vi "FieldSweepScans.vi"() -> ()   [LabVIEW 2021]
uses:
  <instrlib>/Zurich Instruments LabOne/Public/Configure/ziSetValueDoubleArray.vi
  <instrlib>/Zurich Instruments LabOne/Public/Configure/ziSetValueDouble.vi
  <instrlib>/Zurich Instruments LabOne/Public/Configure/ziGetValueDemodSampleEx.vi
  <instrlib>/Zurich Instruments LabOne/Zurich Instruments LabOne.lvlib
panel:
  in  "Tab Control 2":enum32{"Measurement OP"}(tab)
  in  "ms time per field OP":dbl=500.0
  in  "Max OP voltage":dbl
  in  "Min OP voltage":dbl
  in  "Delta OP voltage":dbl=0.25
  in  "N.Loops OOP":i32
  in  "N. measures OP":dbl=1.0
  in  "ms time mes. OP":dbl=500.0
  out "Current OOP":cluster{dbl[], dbl[]}(graph)
  in  "Measure OP":bool
  out "Average OOP":cluster{dbl[], dbl[]}(graph)
  out "OP loop":i32
  in  "stop":bool
  in  "Try IP voltage":enum32{"Single Voltage Output"}(tab)
  in  "OP voltage":dbl
  in  "IP voltage":dbl
  in  "In Plane":bool
  in  "Out Plane":bool
  in  "Tab Control":enum32{"Measurement IP"}(tab)
  in  "Measure IP":bool
  in  "ms time mes. IP":dbl=500.0
  in  "Min IP voltage":dbl
  in  "Delta IP voltage":dbl=0.25
  in  "Max IP voltage":dbl
  in  "N. measures IP":dbl=1.0
  in  "ms time per delta":dbl=500.0
  in  "Loops IP":i32
  out "Current IP":cluster{dbl[], dbl[]}(graph)
  out "Updated IP":cluster{dbl[], dbl[]}(graph)
  out "IP loop":i32
  in  "Lock-In Parameters Tab":enum32{"Lock-In Parameters IP"}(tab)
  in  "Frequency (Hz)":dbl=1092.0
  in  "Harm.":u32=1
  in  "Order 1":enum16{"1", "2", "3", "4", "5", "6", "7", "8"}(ring)=enum."6" caption="Order"
  in  "TC Value 1":dbl=68.99 caption="Value (s/Hz)" format="%#_8g"
  in  "TC/BW 1":enum16{"TC", "BW 3dB"}(ring)=enum."BW 3dB" caption="TC/BW"
  in  "Vpeak (V)":dbl
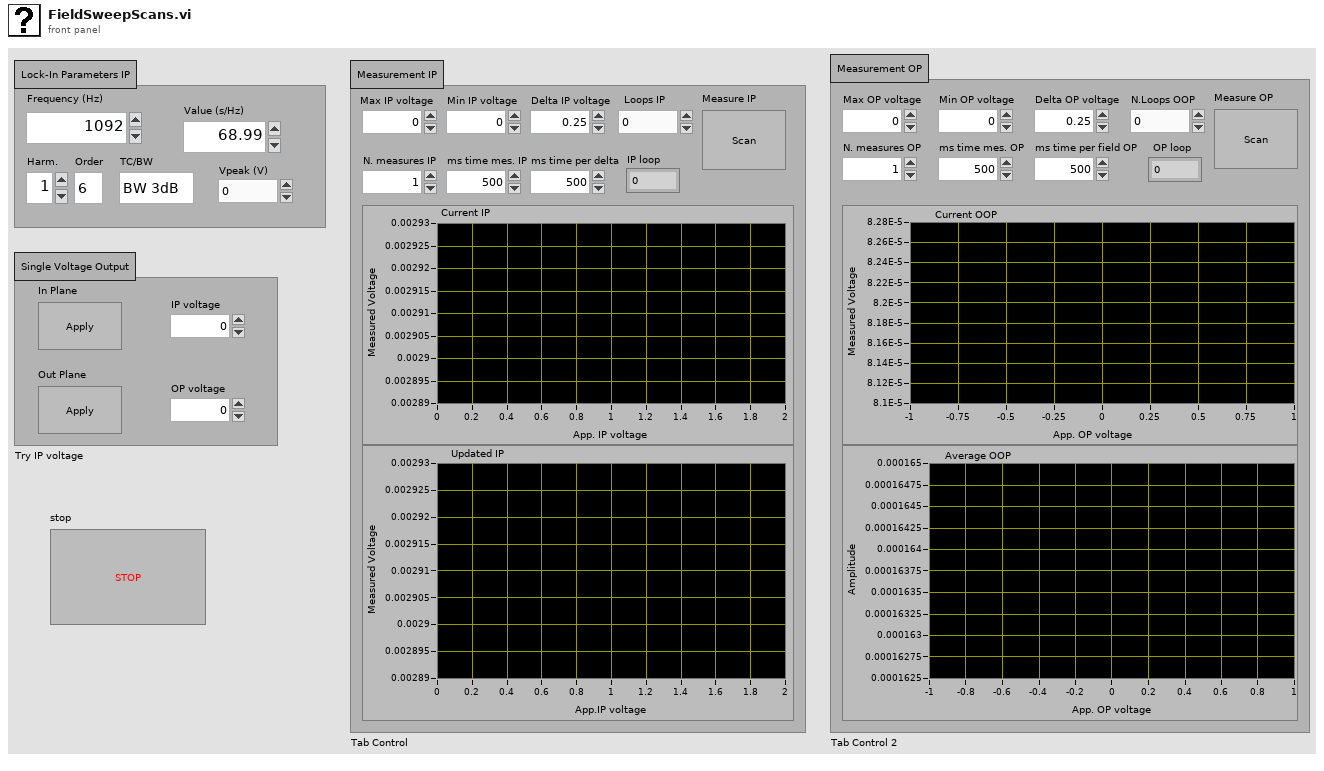
[diagram p1: front panel]
types:
  T1 = typedef "Zurich Instruments LabOne.lvlib/ziTypeHandle.ctl" = cluster{"handleValid":bool, "Conn":u64, "Path Prefix":string, "Handle":u64, "Connected":bool, "Clockbase(s)":dbl}
  T2 = typedef "Zurich Instruments LabOne.lvlib/ziTypeDemodSampleSingle.ctl" = cluster{"Timestamps (ticks)":u64, "X (Vrms)":dbl, "Y (Vrms)":dbl, "Osc Phase (deg)":dbl, "Freq (Hz)":dbl, "DIO":u32, "AuxIn0 (V)":dbl, "AuxIn1 (V)":dbl, "Trigger":u32}
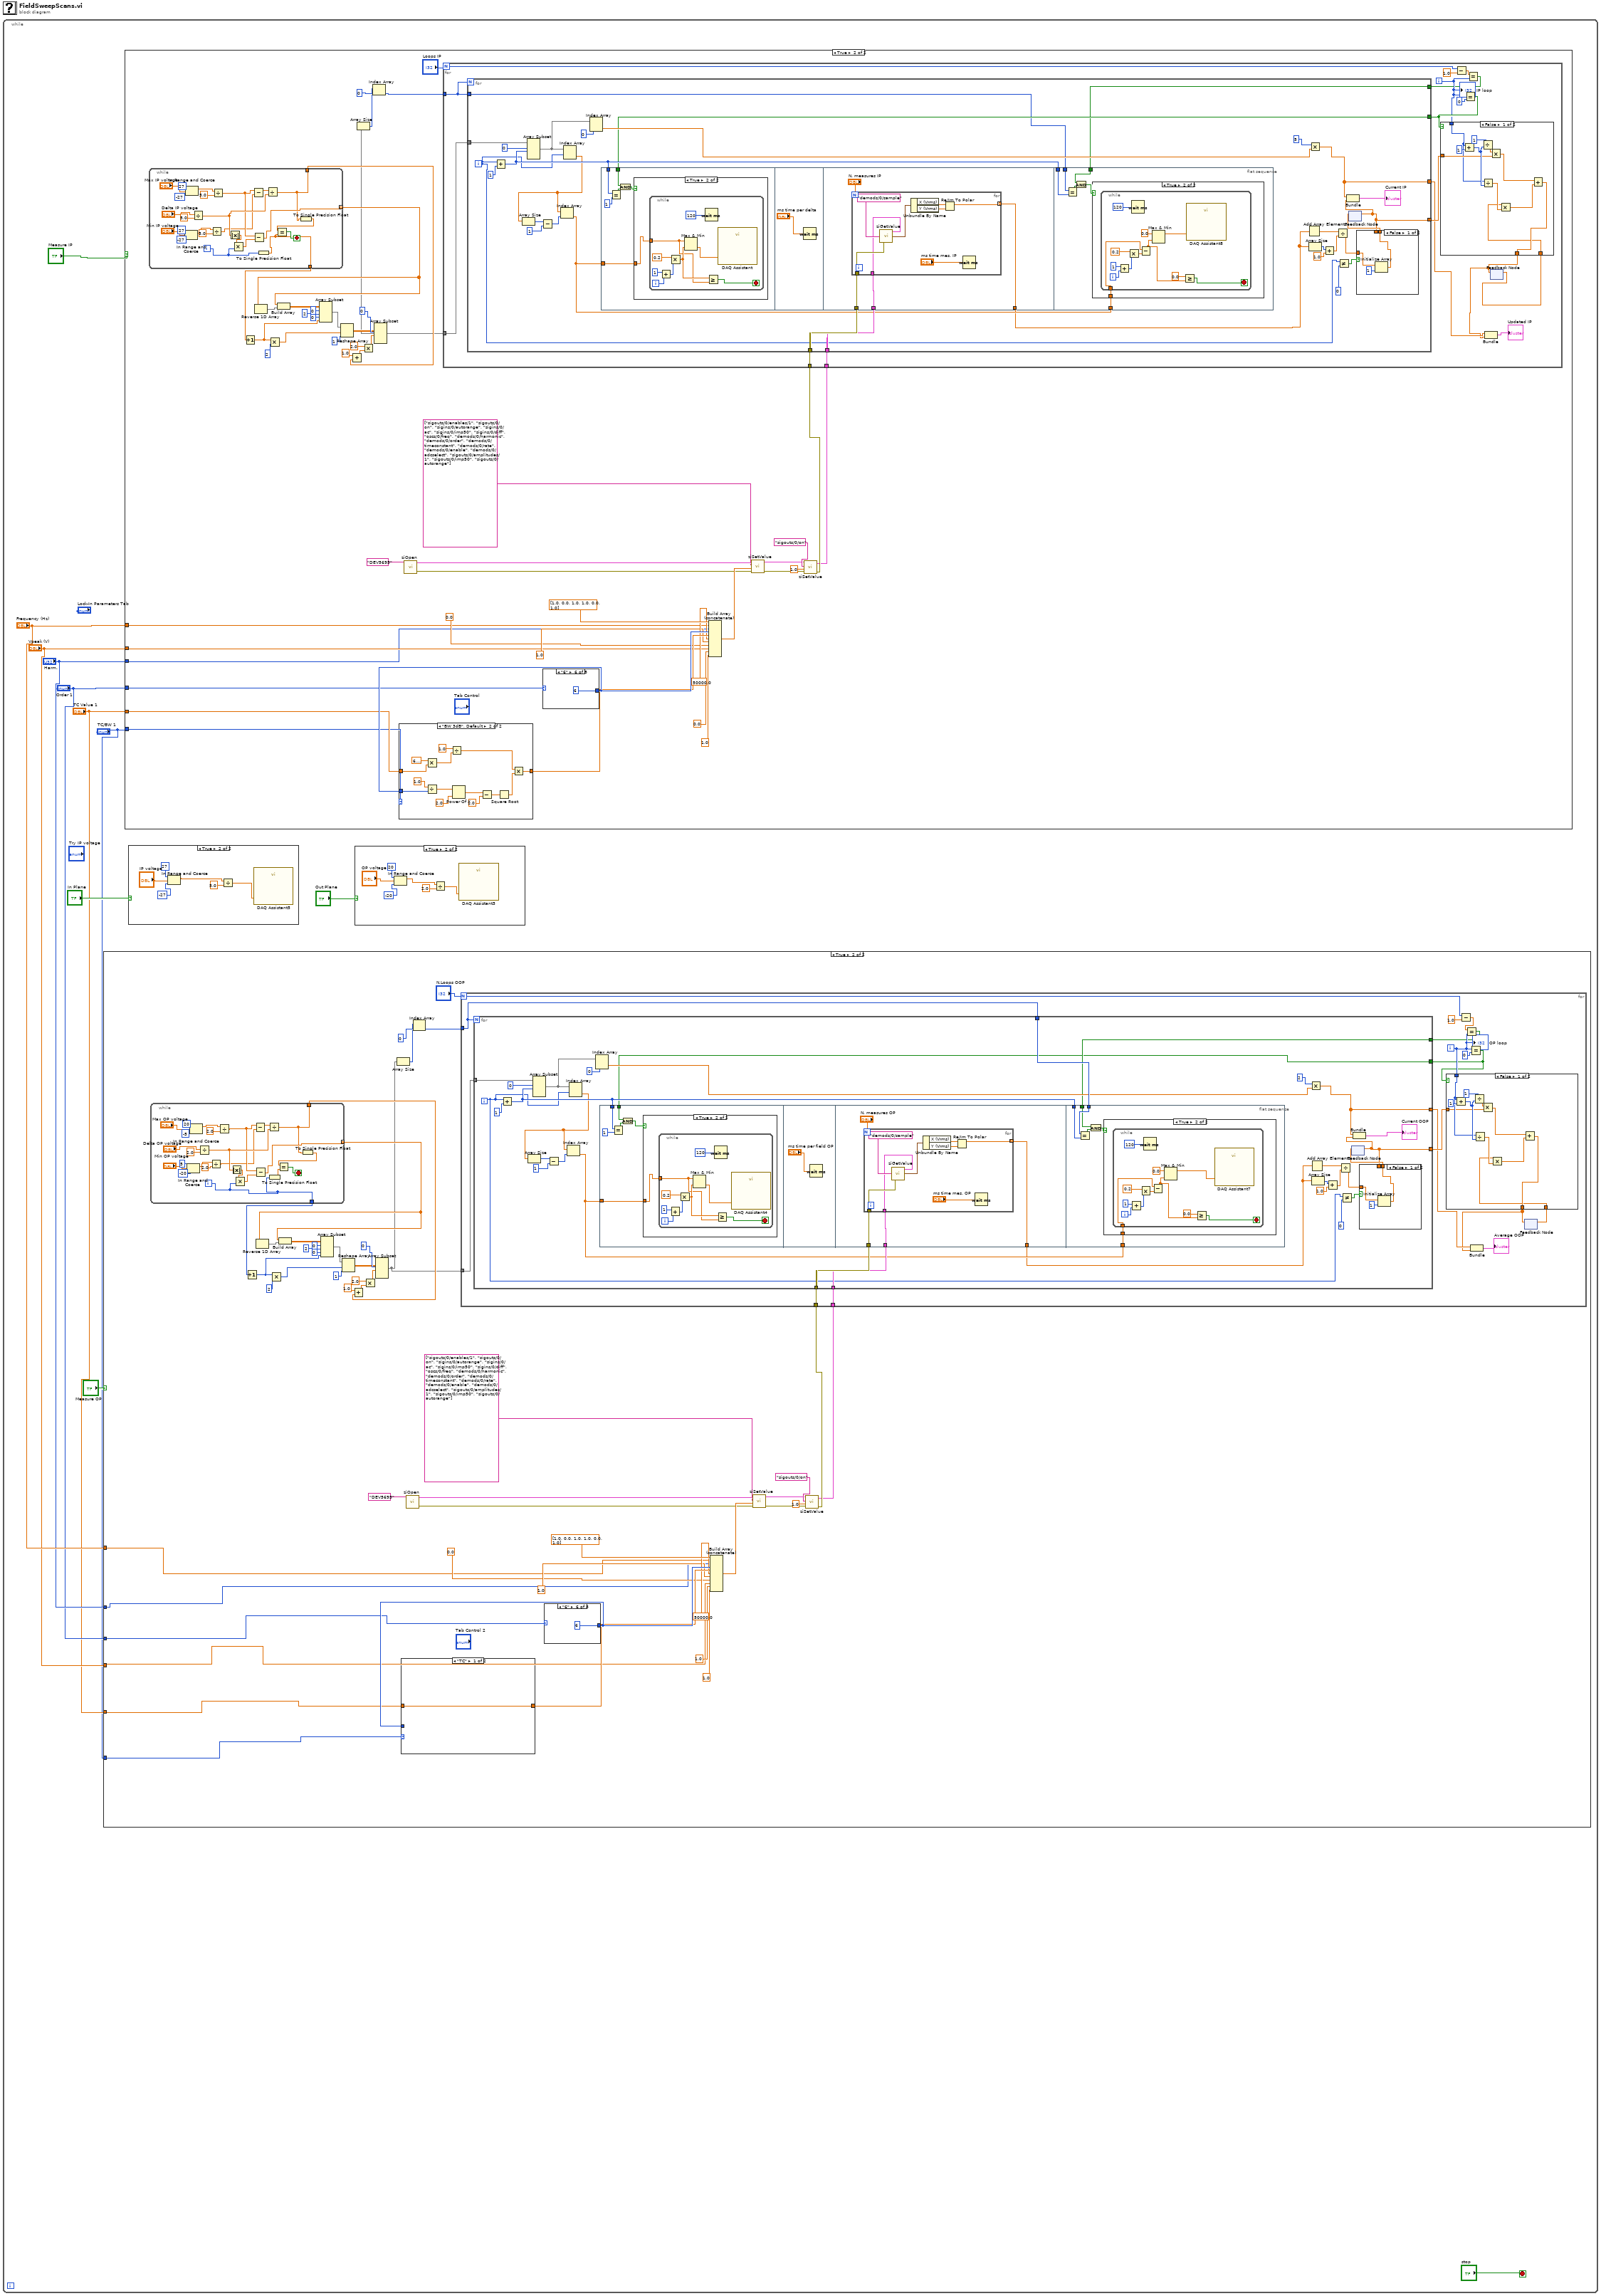
[diagram p0: block diagram]
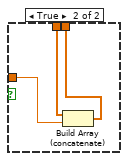
[diagram p4: hidden frame]
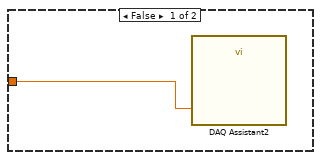
[diagram p5: hidden frame]
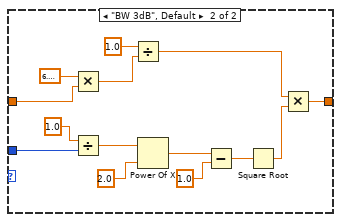
[diagram p7: hidden frame]
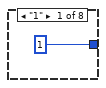
[diagram p8: hidden frame]
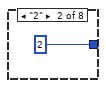
[diagram p9: hidden frame]
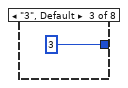
[diagram p10: hidden frame]
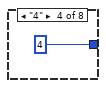
[diagram p11: hidden frame]
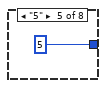
[diagram p12: hidden frame]
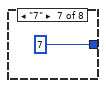
[diagram p13: hidden frame]
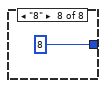
[diagram p14: hidden frame]
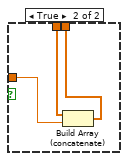
[diagram p19: hidden frame]
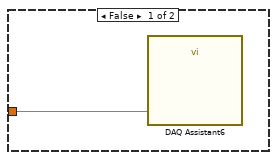
[diagram p20: hidden frame]
diagram:
  n1 = while {
    stop <- "stop" stop-if-true
    n2 = case shown="True" "Measure OP" {
      tunnel: "Frequency (Hz)" -> [_ w18]
      tunnel: "Vpeak (V)" -> [_ w17]
      tunnel: "Harm." -> [_ w16]
      tunnel: "Order 1" -> [_ w15]
      tunnel: "TC Value 1" -> [_ w14]
      tunnel: "TC/BW 1" -> [_ w13]
      frame False {
      }
      frame True {
        n3 = while {
          tunnel: [w194] -> w41 mode=indexing
          tunnel: [w178] -> w38
          tunnel: [w177] -> w33
          i -> [w178]
          stop <- w197 stop-if-true
          n4 = In Range and Coerce(upper limit=5, x="Min OP voltage", lower limit=-20) -> (coerced(x)=w181:dbl)  [unwired: 1 out]
          n5 = In Range and Coerce(upper limit=20, x="Max OP voltage", lower limit=-5) -> (coerced(x)=w183:dbl)  [unwired: 1 out]
          n6 = Divide(x="Delta OP voltage", y=2.0) -> (x/y=w189:dbl)
          n7 = Divide(x=w181, y=2.0) -> (x/y=w179:dbl)
          n8 = Divide(x=w183, y=2.0) -> (x/y=w180:dbl)
          n9 = Absolute Value(x=w189) -> (abs(x)=w196:dbl)
          n10 = Multiply(x=w196, y=w178) -> (x*y=w195:dbl)
          n11 = Subtract(x=w180, y=w179) -> (x-y=w198:dbl)
          n12 = Subtract(x=w180, y=w195) -> (x-y=w194:dbl)
          n13 = Divide(x=w198, y=w189) -> (x/y=w177:dbl)
          n14 = To Single Precision Float(number=w178) -> (single precision float=w176:sgl)
          n15 = To Single Precision Float(number=w177) -> (single precision float=w175:sgl)
          n16 = Equal?(x=w175, y=w176) -> (x = y?=w197:bool)
        }
        n17 = Increment(x=w38) -> (x+1=w22:i32)
        n18 = Reverse 1D Array(array=w41) -> (reversed array=w40:dbl[])
        n19 = Multiply(x=w22, y=2) -> (x*y=w24:i32)
        n20 = Build Array "Build Array"(w41, w40) -> (w21:dbl[][])
        n21 = Array Subset(array=w21, index (row)=0 ("index"), length (row)=2 ("length"), index (col)=0 ("index"), length (col)=w22) -> (w20:dbl[][])
        n22 = Reshape Array(w20, w24, 1 ("dimension size")) -> (w27:dbl[][])
        n23 = Add(x=1.0, y=w33) -> (x+y=w31:dbl)
        n24 = Multiply(x=2.0, y=w31) -> (x*y=w30:dbl)
        n25 = Array Subset(array=w27, index (row)=0 ("index"), length (row)=w30) -> (w28:dbl[][])  [unwired: 2 in]
        n26 = Array Size(array=w28) -> (size(s)=w35:i32[])
        n27 = call <instrlib>:"ziOpen.vi"("Address"="DEV5695") -> ("Error Out"=w57:errorcluster, "HandleOut"=w56:T1)  [unwired: 3 in, 1 out]
        n28 = Index Array(array=w35, index=0) -> (element=w12:i32)
        n29 = case shown="\"6\"" w15 {
          tunnel: [1 2 3 4 5 6 7 8] -> w59
          frame "1" {
          }
          frame "2" {
          }
          frame "3", Default {
          }
          frame "4" {
          }
          frame "5" {
          }
          frame "6" {
          }
          frame "7" {
          }
          frame "8" {
          }
        }
        n30 = case shown="\"TC\"" w13 {
          tunnel: w14 -> [w199 w202]
          tunnel: [w199 w201] -> w58
          tunnel: w59 -> [_ w200]
          frame "TC" {
          }
          frame "BW 3dB", Default {
            n31 = Multiply(x=6.283185307179586, y=w202) -> (x*y=w211:dbl)
            n32 = Divide(x=1.0, y=w200) -> (x/y=w204:dbl)
            n33 = Divide(x=1.0, y=w211) -> (x/y=w208:dbl)
            n34 = Power Of X(1:2.0 ("x"), 2:w204) -> (0:w205:dbl)
            n35 = Subtract(x=w205, y=1.0) -> (x-y=w209:dbl)
            n36 = Square Root(x=w209) -> (sqrt(x)=w207:dbl)
            n37 = Multiply(x=w208, y=w207) -> (x*y=w201:dbl)
          }
        }
        n38 = Build Array (concatenate) "Build Array"(dbl[] [1.0, 0.0, 1.0, 1.0, 0.0, 1.0], w18, w16, w59, w58, 50000.0 ("t"), 1.0 ("t"), 0.0 ("element"), w17, 1.0 ("element"), 1.0 ("element")) -> (w60:dbl[])
        n39 = call-poly <instrlib>:"ziSetValue.vi"("Error In"=w57, "Values"=w60, "Paths"=string[] ["sigouts/0/enables/1", "sigouts/0/on", "sigins/0/autorange", "sigins/0/ac", "sigins/0/imp50", "sigins/0/diff", "oscs/0/freq", "demods/0/harmonic", "demods/0/order", "demods/0/timeconstant", "demods/0/rate", "demods/0/enable", "demods/0/adcselect", "sigouts/0/amplitudes/1", "sigouts/0/imp50", "sigouts/0/autorange"], "Handle In"=w56) -> ("Error Out"=w44:errorcluster, "Handle Out"=w45:T1)  [unwired: 1 in]
        n40 = call-poly <instrlib>:"ziSetValue.vi"("Error In"=w44, "Value"=1.0, "Path"="sigouts/0/on", "Handle In"=w45) -> ("Error Out"=w43:errorcluster, "Handle Out"=w42:T1)  [unwired: 1 in]
        n41 = for {
          N: "N.Loops OOP" -> [w69]
          tunnel: w43 -> [w76]
          tunnel: w42 -> [w75]
          tunnel: w12 -> [w73]
          tunnel: w28 -> [w74]
          i -> [w68]
          n42 = Subtract(x=w69, y=1.0) -> (x-y=w67:dbl)
          n43 = Equal?(x=w67, y=w68) -> (x = y?=w66:bool)
          n44 = Equal?(x=w68, y=0) -> (x = y?=w61:bool)
          n45 = for {
            N: w73 -> [_]
            tunnel: w76 -> [w119]
            tunnel: w75 -> [w118]
            tunnel: w74 -> [w115]
            tunnel: w73 -> [w114]
            tunnel: [w92] -> w64
            tunnel: [w91] -> w65
            tunnel: w66 -> [w90]
            tunnel: w61 -> [w89]
            i -> [w96]
            n46 = Add(x=w96, y=1) -> (x+y=w113:i32)
            n47 = Array Subset(array=w115, index (row)=0 ("index"), length (row)=w113) -> (w106:dbl[][])  [unwired: 2 in]
            n48 = Index Array(array=w106, index (row)=w96) -> (element=w107:dbl[])  [unwired: 1 in]
            n49 = Array Size(array=w107) -> (size(s)=w110:i32)
            n50 = Subtract(x=w110, y=1) -> (x-y=w111:i32)
            n51 = Index Array(array=w107, index=w111) -> (element=w112:dbl)
            n52 = Index Array(array=w106, index (col)=0 ("disabled index (col)")) -> (element=w94:dbl[])  [unwired: 1 in]
            n53 = flat-sequence {
              tunnel: w112 -> [w131]
              tunnel: w113 -> [w130]
              tunnel: w89 -> [w127]
              tunnel: w119 -> [w146]
              tunnel: w118 -> [w145]
              tunnel: [w144] -> w97
              tunnel: w114 -> [w161]
              tunnel: w113 -> [w160]
              tunnel: w112 -> [w159]
              tunnel: w90 -> [w158]
              frame #0 {
                n54 = Equal?(x=w130, y=1) -> (x = y?=w128:bool)
                n55 = And(x=w127, y=w128) -> (x .and. y?=w126:bool)
                n56 = case shown="True" w126 {
                  tunnel: w131 -> [w132 w133]
                  frame False {
                    n57 = call "DAQ Assistant2"("data"=w132) -> ()  [unwired: 17 in, 2 out]
                  }
                  frame True {
                    n58 = while {
                      tunnel: w133 -> [w135]
                      i -> [w142]
                      stop <- w137 stop-if-true
                      n59 = Add(x=1, y=w142) -> (x+y=w140:i32)
                      n60 = Multiply(x=0.2, y=w140) -> (x*y=w136:dbl)
                      n61 = Max & Min(x=w135, y=w136) -> (min(x,y)=w134:dbl)  [unwired: 1 out]
                      n62 = Wait (ms)(milliseconds to wait=u32 120) -> ()  [unwired: 1 out]
                      n63 = Greater Or Equal?(x=w136, y=w135) -> (x >= y?=w137:bool)
                      n64 = call "DAQ Assistant4"("data"=w134) -> ()  [unwired: 17 in, 2 out]
                    }
                  }
                }
              }
              frame #1 {
                n65 = Wait (ms)(milliseconds to wait="ms time per field OP") -> ()  [unwired: 1 out]
              }
              frame #2 {
                n66 = for {
                  N: "N. measures OP" -> [_]
                  tunnel: w146 -> [w151]
                  tunnel: w145 -> [w149]
                  tunnel: [w148] -> w144 mode=indexing
                  n67 = call-poly <instrlib>:"ziGetValue.vi"("error in"=w151, "Path"="demods/0/sample", "Handle In"=w149) -> ("Demod Sample Out"=w152:T2)  [unwired: 2 out]
                  n68 = Unbundle By Name(w152) -> ("X (Vrms)"=w153:dbl, "Y (Vrms)"=w154:dbl)
                  n69 = Re/Im To Polar(2:w154, 3:w153) -> (1:w148:dbl)  [unwired: 1 out]
                  n70 = Wait (ms)(milliseconds to wait="ms time mes. OP") -> ()  [unwired: 1 out]
                }
              }
              frame #3 {
                n71 = Equal?(x=w161, y=w160) -> (x = y?=w157:bool)
                n72 = And(x=w158, y=w157) -> (x .and. y?=w156:bool)
                n73 = case shown="True" w156 {
                  tunnel: w159 -> [_ w162]
                  frame False {
                  }
                  frame True {
                    n74 = while {
                      tunnel: w162 -> [w169]
                      i -> [w170]
                      stop <- w165 stop-if-true
                      n75 = Add(x=1, y=w170) -> (x+y=w172:i32)
                      n76 = Multiply(x=0.2, y=w172) -> (x*y=w168:dbl)
                      n77 = Wait (ms)(milliseconds to wait=u32 120) -> ()  [unwired: 1 out]
                      n78 = Subtract(x=w169, y=w168) -> (x-y=w166:dbl)
                      n79 = Max & Min(x=0.0, y=w166) -> (max(x,y)=w163:dbl)  [unwired: 1 out]
                      n80 = Greater Or Equal?(x=0.0, y=w166) -> (x >= y?=w165:bool)
                      n81 = call "DAQ Assistant7"("data"=w163) -> ()  [unwired: 17 in, 2 out]
                    }
                  }
                }
              }
            }
            n82 = Multiply(x=2, y=w94) -> (x*y=w92:dbl[])
            n83 = Add Array Elements(numeric array=w97) -> (sum=w102:dbl)
            n84 = Array Size(array=w97) -> (size(s)=w103:i32)
            n85 = Add(x=w103, y=1.0) -> (x+y=w101:dbl)
            n86 = Divide(x=w102, y=w101) -> (x/y=w100:dbl)
            n87 = Not Equal?(x=w96, y=0) -> (x != y?=w98:bool)
            n88 = feedback #1() -> (w91:dbl[])  [unwired: 1 in]
            n89 = Bundle(w92, w91) -> (→"Current OOP":cluster{dbl[], dbl[]})  [unwired: 1 in]
            n90 = case shown="False" w98 {
              tunnel: w100 -> [w121 w125]
              tunnel: [w122 w124] -> w95
              tunnel: w91 -> [_ w123]
              frame False {
                n91 = Initialize Array(w121, 1 ("dimension size")) -> (w122:dbl[])
              }
              frame True {
                n92 = Build Array (concatenate)(w123, w125) -> (w124:dbl[])
              }
            }
            n93 = feedback-in #1(w95) -> ()
          }
          n94 = feedback #2() -> (w63:dbl[])  [unwired: 1 in]
          n95 = case shown="False" w61 {
            tunnel: [w83 w88] -> w62
            tunnel: w63 -> [w77 _]
            tunnel: w65 -> [w78 w88]
            tunnel: w68 -> [w79 _]
            frame False {
              n96 = Add(x=w79, y=1) -> (x+y=w82:i32)
              n97 = Divide(x=1, y=w82) -> (x/y=w87:dbl)
              n98 = Divide(x=w79, y=w82) -> (x/y=w86:dbl)
              n99 = Multiply(x=w87, y=w78) -> (x*y=w84:dbl[])
              n100 = Multiply(x=w77, y=w86) -> (x*y=w85:dbl[])
              n101 = Add(x=w84, y=w85) -> (x+y=w83:dbl[])
            }
            frame True {
            }
          }
          n102 = Bundle(w64, w62) -> (→"Average OOP":cluster{dbl[], dbl[]})  [unwired: 1 in]
          n103 = feedback-in #2(w62) -> ()
          "OP loop" <- w68
        }
      }
    }
    n104 = case shown="True" "Measure IP" {
      tunnel: "Vpeak (V)" -> [_ w241]
      tunnel: "Frequency (Hz)" -> [_ w240]
      tunnel: "Harm." -> [_ w239]
      tunnel: "Order 1" -> [_ w238]
      tunnel: "TC Value 1" -> [_ w237]
      tunnel: "TC/BW 1" -> [_ w236]
      frame False {
      }
      frame True {
        n105 = while {
          tunnel: [w416] -> w263 mode=indexing
          tunnel: [w398] -> w260
          tunnel: [w400] -> w255
          i -> [w399]
          stop <- w419 stop-if-true
          n106 = In Range and Coerce(upper limit=27, x="Min IP voltage", lower limit=-27) -> (coerced(x)=w402:dbl)  [unwired: 1 out]
          n107 = In Range and Coerce(upper limit=27, x="Max IP voltage", lower limit=-27) -> (coerced(x)=w407:dbl)  [unwired: 1 out]
          n108 = Divide(x="Delta IP voltage", y=5.0) -> (x/y=w411:dbl)
          n109 = Divide(x=w402, y=5.0) -> (x/y=w401:dbl)
          n110 = Divide(x=w407, y=5.0) -> (x/y=w408:dbl)
          n111 = Absolute Value(x=w411) -> (abs(x)=w418:dbl)
          n112 = Multiply(x=w418, y=w399) -> (x*y=w417:dbl)
          n113 = Subtract(x=w408, y=w401) -> (x-y=w420:dbl)
          n114 = Subtract(x=w408, y=w417) -> (x-y=w416:dbl)
          n115 = To Single Precision Float(number=w399) -> (single precision float=w398:sgl)
          n116 = Divide(x=w420, y=w411) -> (x/y=w400:dbl)
          n117 = To Single Precision Float(number=w400) -> (single precision float=w397:sgl)
          n118 = Equal?(x=w397, y=w398) -> (x = y?=w419:bool)
        }
        n119 = Increment(x=w260) -> (x+1=w245:sgl)
        n120 = Reverse 1D Array(array=w263) -> (reversed array=w262:dbl[])
        n121 = Multiply(x=w245, y=2) -> (x*y=w247:sgl)
        n122 = Build Array "Build Array"(w263, w262) -> (w244:dbl[][])
        n123 = Array Subset(array=w244, index (row)=0 ("index"), length (row)=2 ("length"), index (col)=0 ("index"), length (col)=w245) -> (w243:dbl[][])
        n124 = Reshape Array(w243, w247, 1 ("dimension size")) -> (w250:dbl[][])
        n125 = Add(x=1.0, y=w255) -> (x+y=w253:dbl)
        n126 = Multiply(x=2.0, y=w253) -> (x*y=w252:dbl)
        n127 = Array Subset(array=w250, index (row)=0 ("index"), length (row)=w252) -> (w235:dbl[][])  [unwired: 2 in]
        n128 = Array Size(array=w235) -> (size(s)=w257:i32[])
        n129 = Index Array(array=w257, index=0) -> (element=w234:i32)
        n130 = call <instrlib>:"ziOpen.vi"("Address"="DEV5695") -> ("Error Out"=w279:errorcluster, "HandleOut"=w278:T1)  [unwired: 3 in, 1 out]
        n131 = case shown="\"6\"" w238 {
          tunnel: [1 2 3 4 5 6 7 8] -> w281
          frame "1" {
          }
          frame "2" {
          }
          frame "3", Default {
          }
          frame "4" {
          }
          frame "5" {
          }
          frame "6" {
          }
          frame "7" {
          }
          frame "8" {
          }
        }
        n132 = case shown="\"BW 3dB\", Default" w236 {
          tunnel: w237 -> [w421 w424]
          tunnel: [w421 w423] -> w280
          tunnel: w281 -> [_ w422]
          frame "TC" {
          }
          frame "BW 3dB", Default {
            n133 = Multiply(x=6.283185307179586, y=w424) -> (x*y=w433:dbl)
            n134 = Divide(x=1.0, y=w422) -> (x/y=w426:dbl)
            n135 = Divide(x=1.0, y=w433) -> (x/y=w430:dbl)
            n136 = Power Of X(1:2.0 ("x"), 2:w426) -> (0:w427:dbl)
            n137 = Subtract(x=w427, y=1.0) -> (x-y=w431:dbl)
            n138 = Square Root(x=w431) -> (sqrt(x)=w429:dbl)
            n139 = Multiply(x=w430, y=w429) -> (x*y=w423:dbl)
          }
        }
        n140 = Build Array (concatenate) "Build Array"(dbl[] [1.0, 0.0, 1.0, 1.0, 0.0, 1.0], w240, w239, w281, w280, 50000.0 ("t"), 1.0 ("t"), 0.0 ("element"), w241, 0.0 ("element"), 1.0 ("element")) -> (w282:dbl[])
        n141 = call-poly <instrlib>:"ziSetValue.vi"("Error In"=w279, "Values"=w282, "Paths"=string[] ["sigouts/0/enables/1", "sigouts/0/on", "sigins/0/autorange", "sigins/0/ac", "sigins/0/imp50", "sigins/0/diff", "oscs/0/freq", "demods/0/harmonic", "demods/0/order", "demods/0/timeconstant", "demods/0/rate", "demods/0/enable", "demods/0/adcselect", "sigouts/0/amplitudes/1", "sigouts/0/imp50", "sigouts/0/autorange"], "Handle In"=w278) -> ("Error Out"=w266:errorcluster, "Handle Out"=w267:T1)  [unwired: 1 in]
        n142 = call-poly <instrlib>:"ziSetValue.vi"("Error In"=w266, "Value"=1.0, "Path"="sigouts/0/on", "Handle In"=w267) -> ("Error Out"=w265:errorcluster, "Handle Out"=w264:T1)  [unwired: 1 in]
        n143 = for {
          N: "Loops IP" -> [w290]
          tunnel: w265 -> [w298]
          tunnel: w264 -> [w297]
          tunnel: w235 -> [w296]
          tunnel: w234 -> [w283]
          i -> [w292]
          n144 = Subtract(x=w290, y=1.0) -> (x-y=w289:dbl)
          n145 = Equal?(x=w292, y=0) -> (x = y?=w293:bool)
          n146 = Equal?(x=w289, y=w292) -> (x = y?=w288:bool)
          n147 = for {
            N: w283 -> [_]
            tunnel: w298 -> [w341]
            tunnel: w297 -> [w340]
            tunnel: w296 -> [w337]
            tunnel: [w316] -> w285
            tunnel: [w315] -> w287
            tunnel: w293 -> [w314]
            tunnel: w283 -> [w313]
            tunnel: w288 -> [w312]
            i -> [w319]
            n148 = Add(x=w319, y=1) -> (x+y=w336:i32)
            n149 = Array Subset(array=w337, index (row)=0 ("index"), length (row)=w336) -> (w311:dbl[][])  [unwired: 2 in]
            n150 = Index Array(array=w311, index (row)=w319) -> (element=w331:dbl[])  [unwired: 1 in]
            n151 = Array Size(array=w331) -> (size(s)=w333:i32)
            n152 = Subtract(x=w333, y=1) -> (x-y=w334:i32)
            n153 = Index Array(array=w331, index=w334) -> (element=w335:dbl)
            n154 = Index Array(array=w311, index (col)=0 ("disabled index (col)")) -> (element=w317:dbl[])  [unwired: 1 in]
            n155 = flat-sequence {
              tunnel: w335 -> [w353]
              tunnel: w336 -> [w352]
              tunnel: w314 -> [w349]
              tunnel: w341 -> [w368]
              tunnel: w340 -> [w367]
              tunnel: [w366] -> w320
              tunnel: w313 -> [w383]
              tunnel: w336 -> [w382]
              tunnel: w335 -> [w381]
              tunnel: w312 -> [w379]
              frame #0 {
                n156 = Equal?(x=w352, y=1) -> (x = y?=w348:bool)
                n157 = And(x=w349, y=w348) -> (x .and. y?=w350:bool)
                n158 = case shown="True" w350 {
                  tunnel: w353 -> [w354 w355]
                  frame False {
                    n159 = call "DAQ Assistant6"("data"=w354) -> ()  [unwired: 17 in, 2 out]
                  }
                  frame True {
                    n160 = while {
                      tunnel: w355 -> [w356]
                      i -> [w364]
                      stop <- w358 stop-if-true
                      n161 = Add(x=1, y=w364) -> (x+y=w362:i32)
                      n162 = Multiply(x=0.2, y=w362) -> (x*y=w357:dbl)
                      n163 = Max & Min(x=w356, y=w357) -> (min(x,y)=w359:dbl)  [unwired: 1 out]
                      n164 = Wait (ms)(milliseconds to wait=u32 120) -> ()  [unwired: 1 out]
                      n165 = Greater Or Equal?(x=w357, y=w356) -> (x >= y?=w358:bool)
                      n166 = call "DAQ Assistant"("data"=w359) -> ()  [unwired: 17 in, 2 out]
                    }
                  }
                }
              }
              frame #1 {
                n167 = Wait (ms)(milliseconds to wait="ms time per delta") -> ()  [unwired: 1 out]
              }
              frame #2 {
                n168 = for {
                  N: "N. measures IP" -> [_]
                  tunnel: w368 -> [w373]
                  tunnel: w367 -> [w371]
                  tunnel: [w370] -> w366 mode=indexing
                  n169 = call-poly <instrlib>:"ziGetValue.vi"("error in"=w373, "Path"="demods/0/sample", "Handle In"=w371) -> ("Demod Sample Out"=w374:T2)  [unwired: 2 out]
                  n170 = Unbundle By Name(w374) -> ("X (Vrms)"=w375:dbl, "Y (Vrms)"=w376:dbl)
                  n171 = Re/Im To Polar(2:w376, 3:w375) -> (1:w370:dbl)  [unwired: 1 out]
                  n172 = Wait (ms)(milliseconds to wait="ms time mes. IP") -> ()  [unwired: 1 out]
                }
              }
              frame #3 {
                n173 = Equal?(x=w383, y=w382) -> (x = y?=w378:bool)
                n174 = And(x=w379, y=w378) -> (x .and. y?=w380:bool)
                n175 = case shown="True" w380 {
                  tunnel: w381 -> [_ w384]
                  frame False {
                  }
                  frame True {
                    n176 = while {
                      tunnel: w384 -> [w391]
                      i -> [w392]
                      stop <- w386 stop-if-true
                      n177 = Add(x=1, y=w392) -> (x+y=w394:i32)
                      n178 = Multiply(x=0.2, y=w394) -> (x*y=w390:dbl)
                      n179 = Wait (ms)(milliseconds to wait=u32 120) -> ()  [unwired: 1 out]
                      n180 = Subtract(x=w391, y=w390) -> (x-y=w387:dbl)
                      n181 = Max & Min(x=0.0, y=w387) -> (max(x,y)=w388:dbl)  [unwired: 1 out]
                      n182 = Greater Or Equal?(x=0.0, y=w387) -> (x >= y?=w386:bool)
                      n183 = call "DAQ Assistant8"("data"=w388) -> ()  [unwired: 17 in, 2 out]
                    }
                  }
                }
              }
            }
            n184 = Add Array Elements(numeric array=w320) -> (sum=w327:dbl)
            n185 = Array Size(array=w320) -> (size(s)=w328:i32)
            n186 = Multiply(x=5, y=w317) -> (x*y=w316:dbl[])
            n187 = Add(x=w328, y=1.0) -> (x+y=w326:dbl)
            n188 = Divide(x=w327, y=w326) -> (x/y=w325:dbl)
            n189 = Not Equal?(x=w319, y=0) -> (x != y?=w323:bool)
            n190 = feedback #3() -> (w315:dbl[])  [unwired: 1 in]
            n191 = Bundle(w316, w315) -> (→"Current IP":cluster{dbl[], dbl[]})  [unwired: 1 in]
            n192 = case shown="False" w323 {
              tunnel: w325 -> [w343 w347]
              tunnel: [w344 w346] -> w322
              tunnel: w315 -> [_ w345]
              frame False {
                n193 = Initialize Array(w343, 1 ("dimension size")) -> (w344:dbl[])
              }
              frame True {
                n194 = Build Array (concatenate)(w345, w347) -> (w346:dbl[])
              }
            }
            n195 = feedback-in #3(w322) -> ()
          }
          n196 = feedback #4() -> (w286:dbl[])  [unwired: 1 in]
          n197 = case shown="False" w293 {
            tunnel: [w302 w310] -> w284
            tunnel: w286 -> [w301 _]
            tunnel: w287 -> [w300 w310]
            tunnel: w292 -> [w299 _]
            frame False {
              n198 = Add(x=w299, y=1) -> (x+y=w305:i32)
              n199 = Divide(x=1, y=w305) -> (x/y=w309:dbl)
              n200 = Divide(x=w299, y=w305) -> (x/y=w308:dbl)
              n201 = Multiply(x=w309, y=w300) -> (x*y=w306:dbl[])
              n202 = Multiply(x=w301, y=w308) -> (x*y=w307:dbl[])
              n203 = Add(x=w306, y=w307) -> (x+y=w302:dbl[])
            }
            frame True {
            }
          }
          n204 = Bundle(w285, w284) -> (→"Updated IP":cluster{dbl[], dbl[]})  [unwired: 1 in]
          n205 = feedback-in #4(w284) -> ()
          "IP loop" <- w292
        }
      }
    }
    n206 = case shown="True" "In Plane" {
      frame False {
      }
      frame True {
        n207 = In Range and Coerce(upper limit=27, x="IP voltage", lower limit=-27) -> (coerced(x)=w223:dbl)  [unwired: 1 out]
        n208 = Divide(x=w223, y=5.0) -> (x/y=w222:dbl)
        n209 = call "DAQ Assistant5"("data"=w222) -> ()  [unwired: 17 in, 2 out]
      }
    }
    n210 = case shown="True" "Out Plane" {
      frame False {
      }
      frame True {
        n211 = In Range and Coerce(upper limit=20, x="OP voltage", lower limit=-20) -> (coerced(x)=w229:dbl)  [unwired: 1 out]
        n212 = Divide(x=w229, y=2.0) -> (x/y=w228:dbl)
        n213 = call "DAQ Assistant3"("data"=w228) -> ()  [unwired: 17 in, 2 out]
      }
    }
  }
